vi "Day 11-1.vi"() -> ()   [LabVIEW 2019, in "Day 11.lvlib"]
uses:
  Day 11.lvlib
panel:
  in  "Steps":i32=100
  out "Array n":i32[][](array[numeric])=[[1, 1, 1, 3, 2, 2, 7, 5, 4, 8], [1, 1, 5, 3, 2, 2, 2, 6, 4, 4], [1, 6, 3, 2, 2, 2, 3, 8, 5, 4], [1, 5, 2, 2, 2, 3, 5, 1, 8, 6], [1, 5, 2, 2, 3, 5, 1, 1, 1, 1], [1, 4, 2, 3, 5, 1, 1, 1, 1, 1], [3, 4, 4, 6, 1, 1, 1, 1, 1, 1], [9, 9, 1, 2, 3, 3, 2, 1, 1, 7], [8, 1, 2, 4, 0, 0, 4, 2, 7, 5], [7, 1, 2, 0, 0, 0, 0, 7, 5, 4]]
  out "Ligths":bool[][](array[boolean])=[[FALSE, FALSE, FALSE, FALSE, FALSE, FALSE, FALSE, FALSE, FALSE, FALSE], [FALSE, FALSE, FALSE, FALSE, FALSE, FALSE, FALSE, FALSE, FALSE, FALSE], [FALSE, FALSE, FALSE, FALSE, FALSE, FALSE, FALSE, FALSE, FALSE, FALSE], [FALSE, FALSE, FALSE, FALSE, FALSE, FALSE, FALSE, FALSE, FALSE, FALSE], [FALSE, FALSE, FALSE, FALSE, FALSE, FALSE, FALSE, FALSE, FALSE, FALSE], [FALSE, FALSE, FALSE, FALSE, FALSE, FALSE, FALSE, FALSE, FALSE, FALSE], [FALSE, FALSE, FALSE, FALSE, FALSE, FALSE, FALSE, FALSE, FALSE, FALSE], [FALSE, FALSE, FALSE, FALSE, FALSE, FALSE, FALSE, FALSE, FALSE, FALSE], [FALSE, FALSE, FALSE, FALSE, TRUE, TRUE, FALSE, FALSE, FALSE, FALSE], [FALSE, FALSE, FALSE, TRUE, TRUE, TRUE, TRUE, FALSE, FALSE, FALSE]]
  out "Flashes":i32=1683
  out "Array n-1":i32[][](array[numeric])=[[0, 0, 0, 2, 1, 1, 6, 4, 3, 7], [0, 0, 4, 2, 1, 1, 1, 5, 3, 3], [0, 5, 2, 1, 1, 1, 2, 7, 4, 3], [0, 4, 1, 1, 1, 2, 4, 0, 7, 5], [0, 4, 1, 1, 2, 4, 0, 0, 0, 0], [0, 3, 1, 2, 4, 0, 0, 0, 0, 0], [2, 3, 3, 5, 0, 0, 0, 0, 0, 0], [8, 8, 0, 0, 0, 0, 0, 0, 0, 6], [7, 0, 0, 0, 9, 9, 0, 0, 6, 4], [6, 0, 0, 8, 6, 6, 8, 5, 4, 3]]
  in  "String":string="8826876714\n3127787238\n8182852861\n4655371483\n3864551365\n1878253581\n8317422437\n1517254266\n2621124761\n3473331514"
  # "1671\ntoo low"
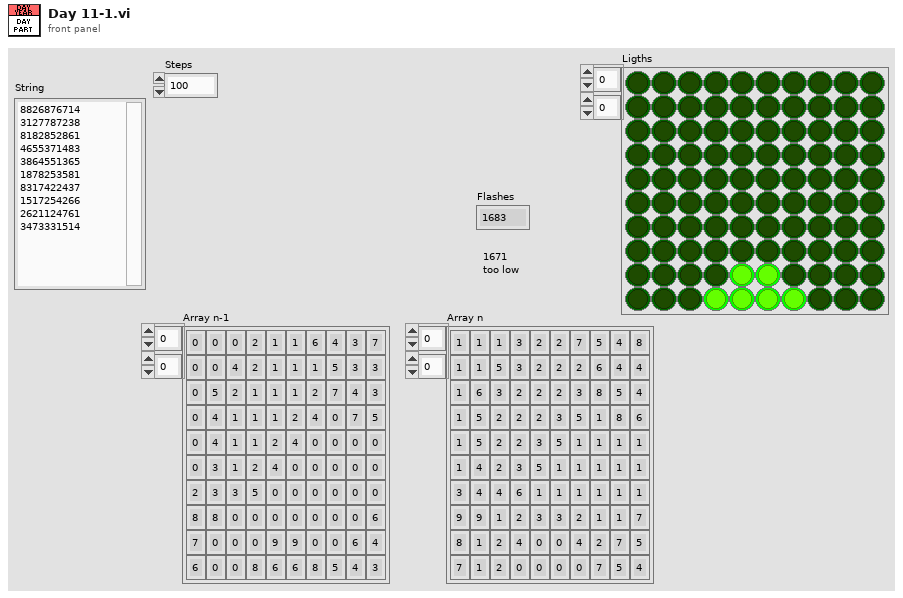
[diagram p1: front panel]
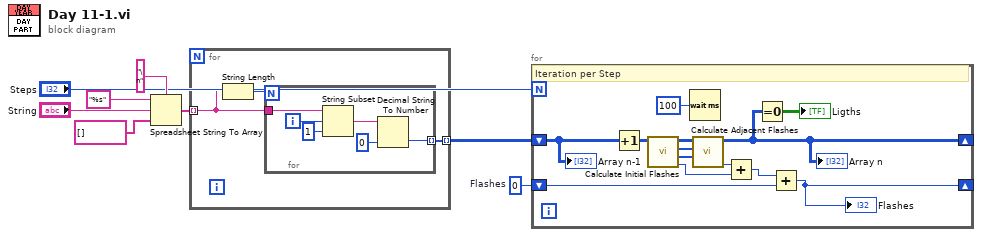
[diagram p0: block diagram]
diagram:
  w2 = 0  # Flashes
  n1 = Spreadsheet String To Array(delimiter (Tab)="\n", format string="%s", spreadsheet string="String", array type (2D Dbl)=string[] []) -> (array=w4:string[])
  n2 = for {
    tunnel: w4 -> [w11] mode=indexing
    tunnel: [w9] -> w3 mode=indexing
    n3 = String Length(string=w11) -> (length=w10:i32)
    n4 = for {
      N: w10 -> [_]
      tunnel: w11 -> [w17]
      tunnel: [w13] -> w9 mode=indexing
      i -> [w16]
      n5 = String Subset(string=w17, offset (0)=w16, length (rest)=1 ("length (rest)")) -> (substring=w14:string)
      n6 = Decimal String To Number(string=w14, default (0L)=0 ("default (0 I32)")) -> (number=w13:i32)  [unwired: 1 in, 1 out]
    }
  }
  n7 = for {
    N: "Steps" -> [_]
    shift-right: [w19] -> _
    shift-left: w3 -> [w20]
    shift-right: [w18] -> _
    shift-left: w2 -> [w23]
    # "Iteration per Step"
    n8 = Increment(x=w20) -> (x+1=w30:i32[][])
    n9 = call "Calculate Initial Flashes.vi"("Octopus Energy Matrix In"=w30) -> ("Flash Count"=w25:i32, "Flashes Columns"=w27:i32[], "Flashes Rows"=w28:i32[], "Octopus Energy Matrix Out"=w29:i32[][])  [unwired: 7 in]
    n10 = Wait (ms)(milliseconds to wait=u32 100) -> ()  [unwired: 1 out]
    n11 = call "Calculate Adjacent Flashes.vi"("Flashes Columns"=w27, "Flashes Rows"=w28, "Octopus Energy Matrix In"=w29) -> ("Flash Count"=w26:i32, "Octopus Energy Matrix Out"=w19:i32[][])  [unwired: 7 in]
    "Array n" <- w19
    n12 = Add(x=w26, y=w25) -> (x+y=w24:i32)
    n13 = Equal To 0?(x=w19) -> (x = 0?=→"Ligths":bool[][])
    n14 = Add(x=w24, y=w23) -> (x+y=w18:i32)
    "Flashes" <- w18
    "Array n-1" <- w20
  }
